vi "Demo.vi"() -> ()   [LabVIEW 2016]
doc: "查看程序详细说明请访问：http://ruanqizhen.spaces.live.com/blog/cns!5852D4F797C53FB6!3382.entry"
uses:
  Othello.xctl
panel:
  out "messege":string
  in  "new":bool
  in  "exit":bool
  in  "Othello":T1[][](xcontrol)
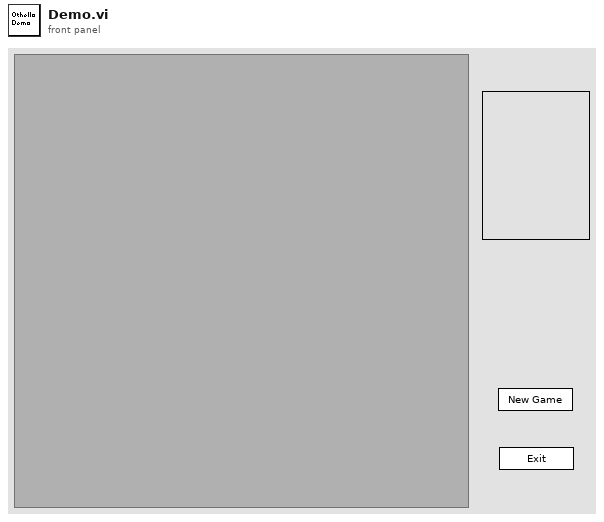
[diagram p1: front panel]
types:
  T1 = typedef "Othello.xctl/Pict Ring Chess.ctl" = u16
  T2 = typedef "Othello.xctl/Interactive Action.ctl" = refnum<user-event>
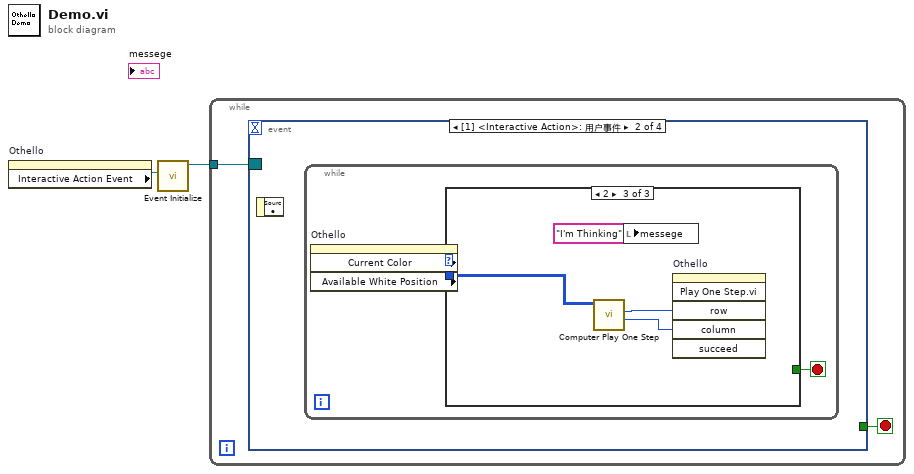
[diagram p0: block diagram]
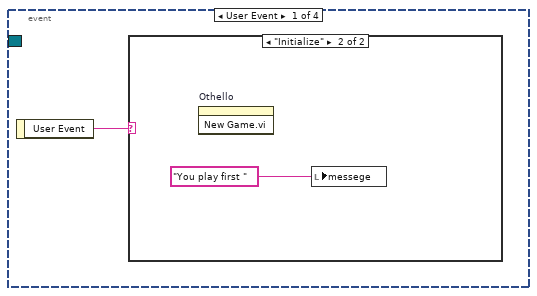
[diagram p2: hidden frame]
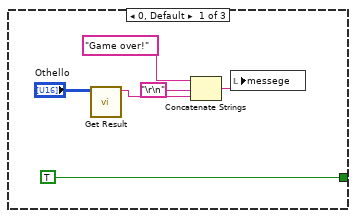
[diagram p4: hidden frame]
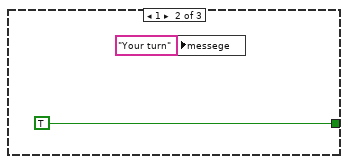
[diagram p5: hidden frame]
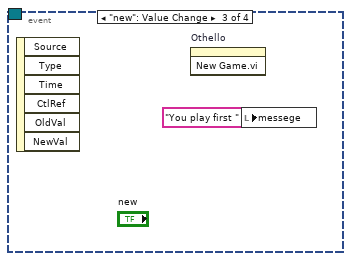
[diagram p6: hidden frame]
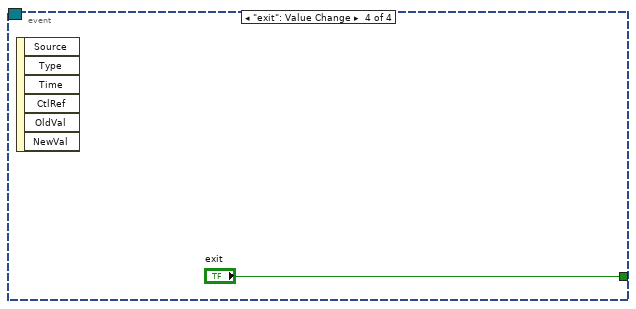
[diagram p7: hidden frame]
diagram:
  n1 = property on="Othello" class="Othello (严格)"() -> ("Interactive Action Event"=w1:T2)  [unwired: 2 in, 2 out]
  n2 = call "Event Initialize.vi"("Interactive Action"=w1) -> ("Event Reg Ref"=w2:refnum<event-registration>)  [unwired: 10 out]
  n3 = while {
    tunnel: w2 -> [w4]
    stop <- w3 stop-if-true
    n4 = event shown="[1] <Interactive Action>: 用户事件" {
      selector: w4 -> [_ _ _ _]
      dyn-events: _ -> [_ _ _ _]
      timeout: _ -> [_ _ _ _]
      tunnel: [_ _ _ "exit"] -> w3
      event User Event {
        n5 = event-data() -> ("User Event"=w5:string)  [unwired: 1 out]
        n6 = case shown="\"Initialize\"" w5 {
          frame "假", Default {
          }
          frame "Initialize" {
            n7 = invoke on="Othello" class="Othello (严格)" method="New Game.vi"() -> ()  [unwired: 3 in, 3 out]
            n8 = local write "messege"("You play first " ("messege")) -> ()
          }
        }
      }
      event User Event {
        n9 = event-data() -> ()  [unwired: 2 out]
        n10 = while {
          stop <- w8 stop-if-true
          n11 = property on="Othello" class="Othello (严格)"() -> ("Current Color"=w9:T1, "Available White Position"=w7:i32[][])  [unwired: 2 in, 2 out]
          n12 = case shown="2" w9 {
            tunnel: [TRUE TRUE _] -> w8
            tunnel: w7 -> [_ _ w20]
            frame 0, Default {
              n13 = call "Get Result.vi"("Othello"="Othello") -> ("Resule"=w13:string)  [unwired: 10 out]
              n14 = Concatenate Strings("Game over!" ("messege"), "\r\n", w13) -> (w11:string)
              n15 = local write "messege"(w11) -> ()
            }
            frame 1 {
              n16 = local write "messege"("Your turn" ("messege")) -> ()
            }
            frame 2 {
              n17 = call "Computer Play One Step.vi"("Available White Position"=w20) -> ("column"=w18:i32, "row"=w19:i32)  [unwired: 1 in, 8 out]
              n18 = local write "messege"("I'm Thinking" ("messege")) -> ()
              n19 = invoke on="Othello" class="Othello (严格)" method="Play One Step.vi"("row"=w19, "column"=w18) -> ()  [unwired: 4 in, 6 out]
            }
          }
        }
      }
      event "new": Value Change {
        n20 = event-data() -> ()  [unwired: 7 out]
        n21 = invoke on="Othello" class="Othello (严格)" method="New Game.vi"() -> ()  [unwired: 3 in, 3 out]
        n22 = local write "messege"("You play first " ("messege")) -> ()
      }
      event "exit": Value Change {
        n23 = event-data() -> ()  [unwired: 7 out]
      }
    }
  }
